vi "read report n write as formate sql.vi"(8 "error in":errorcluster, 10 "Table Name":string="Detailed_Report", 11 "file path (dialog if empty)":path) -> (0 "error out":errorcluster)   [LabVIEW 2017]
uses:
  <vilib>/Utility/file.llb/Read Delimited Spreadsheet (string).vi
panel:
  out "array w/ subset deleted":string[][](array[string])
  out "all rows":string[][](array[string])
  out "Serial Number":string
  in  "User Name 2":string="mmk"
  in  "Shift 2":string="A"
  in  "Test Type 2":string="Test type"
  in  "Excepted Value 2":string="Excepted Value"
  out "Application Verision":string
  out "Variant":string
  out "Model":string
  out "all rows 2":string[][](array[string])
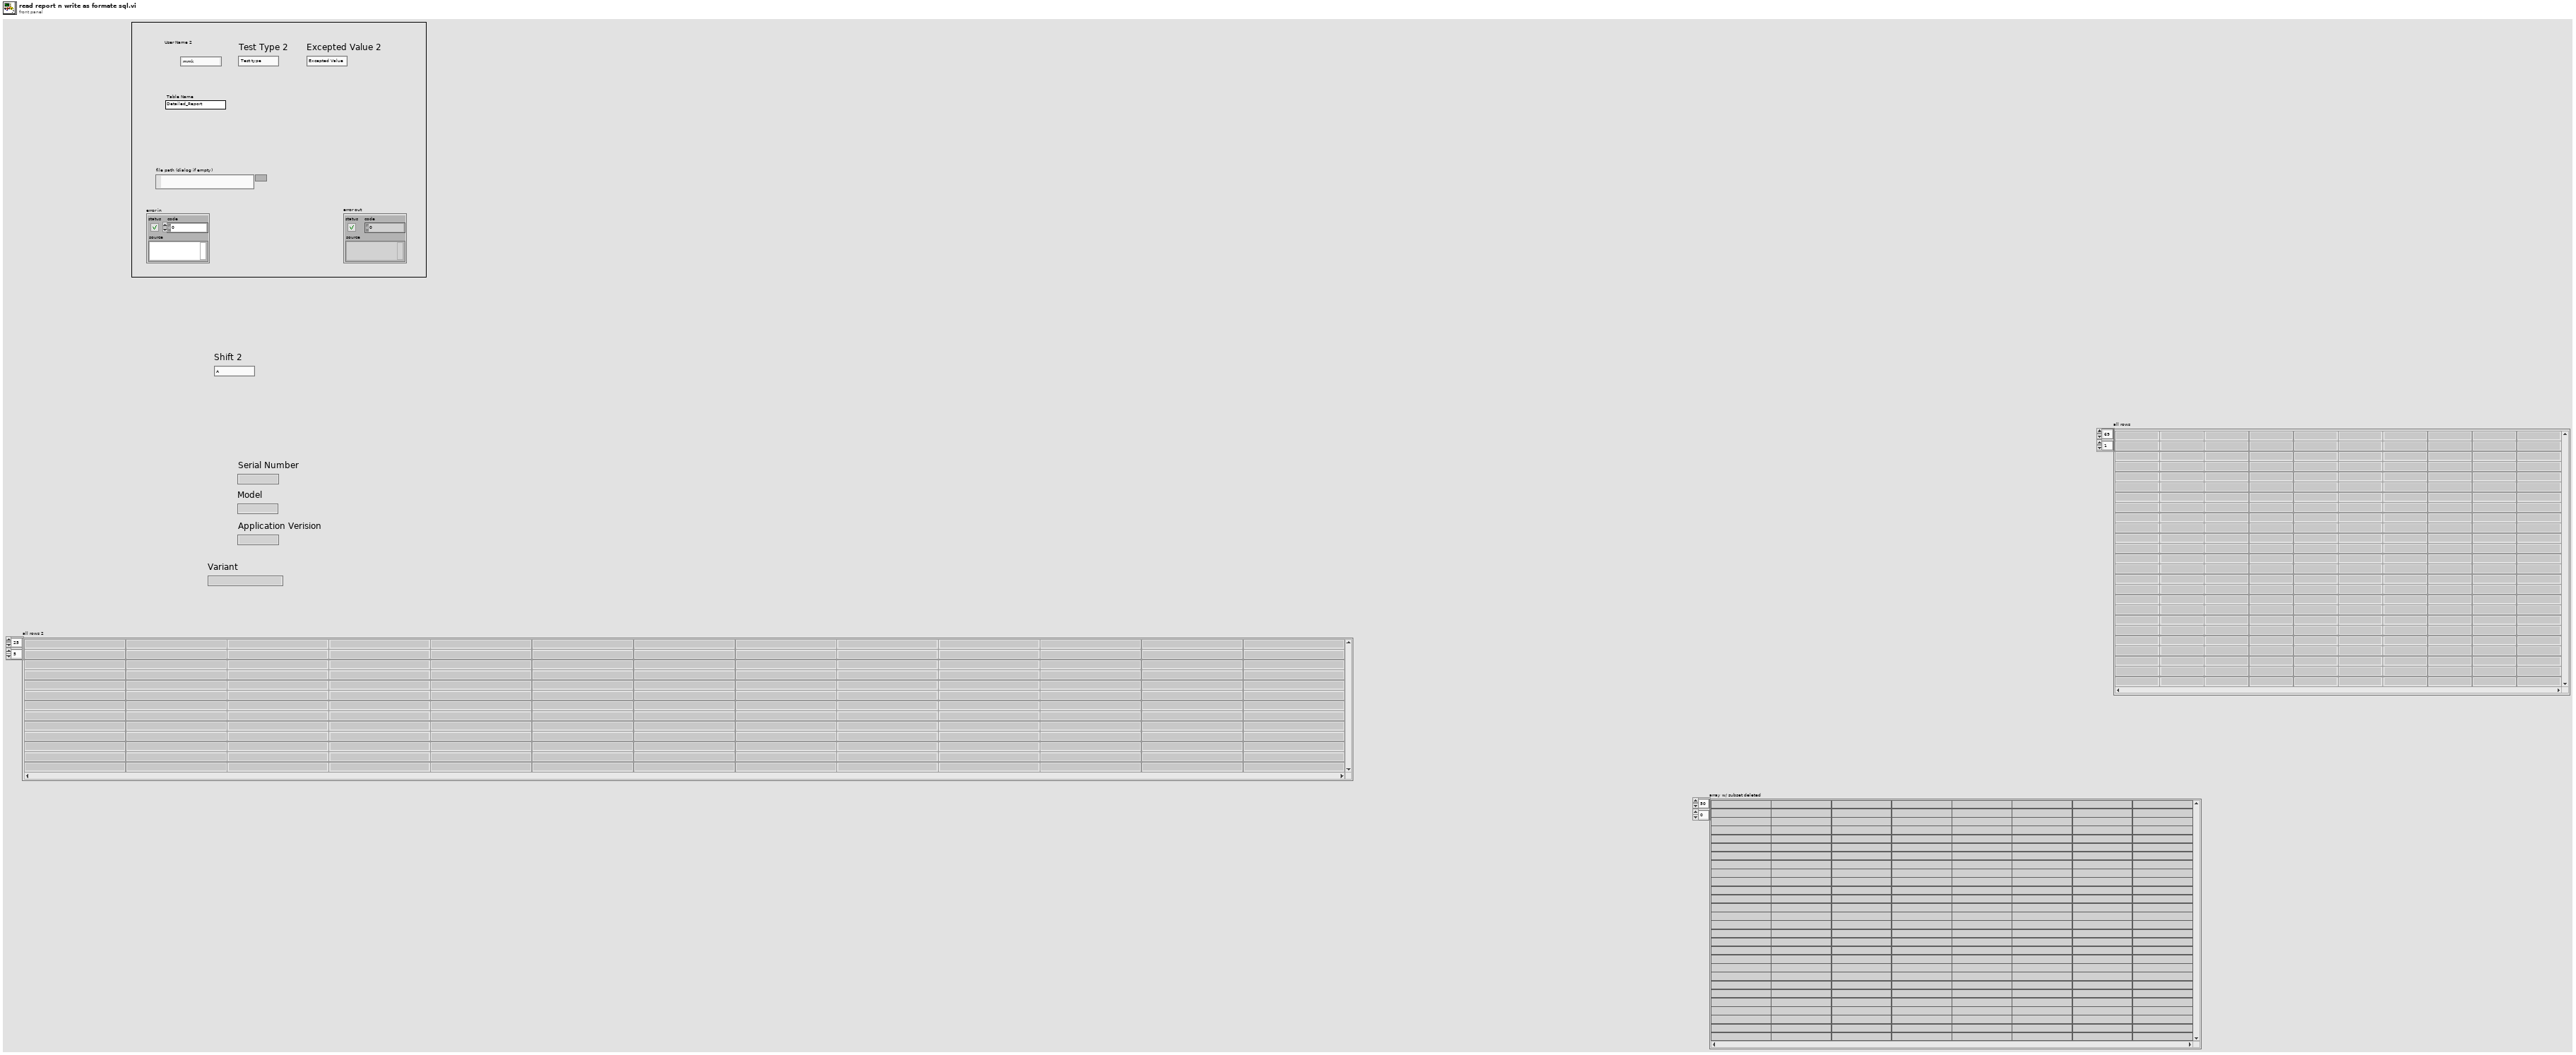
[diagram p1: front panel]
types:
  T1 = cluster{string, string, string, string, string, string, string, string, string, string, string, string, string, string, string}
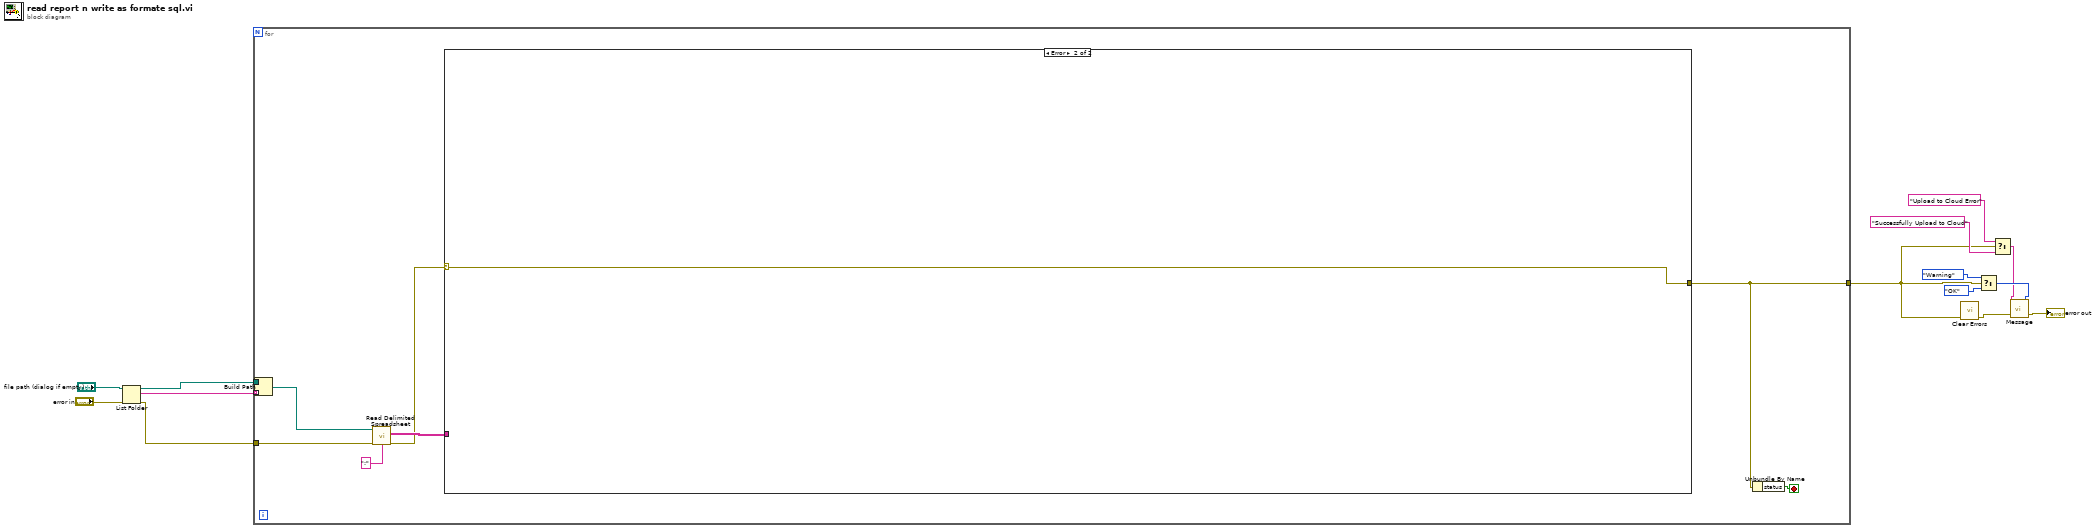
[diagram p0: block diagram]
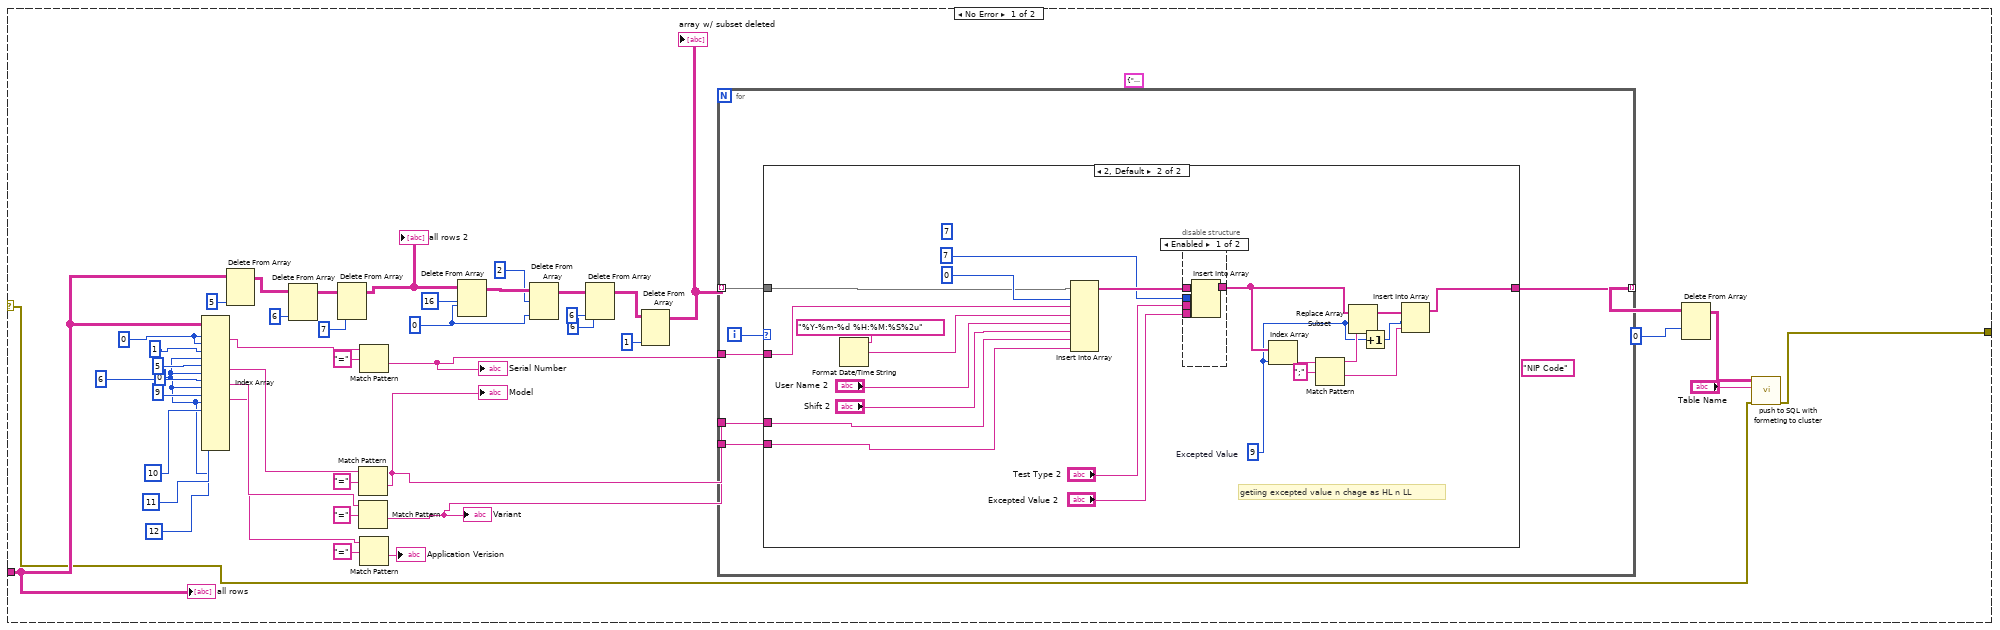
[diagram p2: hidden frame]
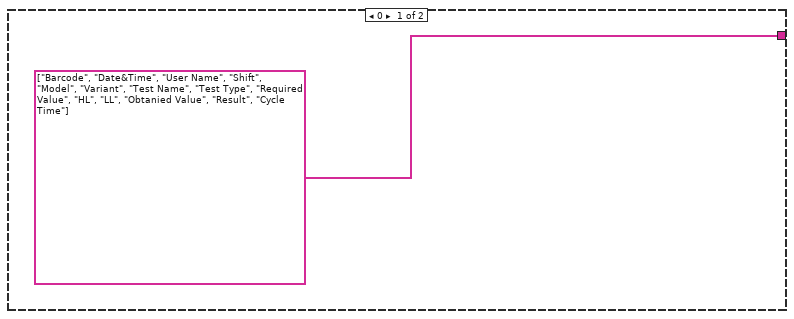
[diagram p3: hidden frame]
diagram:
  n1 = List Folder(path="file path (dialog if empty)", error in="error in") -> (path out=w12:path, filenames=w13:string[], error out=w1:errorcluster)  [unwired: 2 in, 1 out]
  n2 = for {
    tunnel: w13 -> [w19] mode=indexing
    tunnel: w12 -> [w20]
    tunnel: w1 -> [w17]
    tunnel: [w15] -> w6
    stop <- w16 stop-if-true
    n3 = Build Path(base path=w20, name or relative path=w19) -> (appended path=w18:path)
    n4 = call-poly <vilib>:"Read Delimited Spreadsheet.vi"("file path (dialog if empty)"=w18, "error in (no error)"=w17, "delimiter (\\t)"=":" ("delimiter (\\t)")) -> ("all rows"=w22:string[][], "error out"=w21:errorcluster)  [unwired: 7 in, 4 out]
    n5 = case shown="Error" w21 {
      selector: w21 -> [w26 w103]
      tunnel: w22 -> [w41 _]
      tunnel: [w24 w103] -> w15
      frame No Error {
        (unwired) T1 {"barcode", "2019-12-13 20:24:09.05", "1", "shifr", "model", "variant", "test name", "test type", "hl", "ll", "shifr", "obtained", "resrut", "Cycle time", "nip code"}
        w56 = 0 ("index (row)")
        w48 = 0 ("disabled index (col)")
        w37 = 0 ("disabled index (col)")
        n6 = Index Array(array=w41, index (row) #1=w56, index (col) #1=w56, index (row) #2=1 ("index (row)"), index (col) #2=w37, index (row) #3=5 ("index (row)"), index (col) #3=w37, index (row) #4=6 ("index (row)"), index (col) #4=w37, index (row) #5=9 ("index (row)"), index (col) #5=w37, index (row) #6=10 ("index (row)"), index (col) #6=w37, index (row) #7=11 ("index (row)"), index (col) #7=w37, index (row) #8=12 ("index (row)"), index (col) #8=w37) -> (element #1=w54:string, element #3=w66:string, element #4=w63:string, element #5=w59:string)  [unwired: 4 out]
        n7 = Delete From Array(array=w41, index (col)=5 ("disabled index (col)")) -> (array with subset deleted=w40:string[][])  [unwired: 2 in, 1 out]
        n8 = Delete From Array(array=w40, index (col)=6 ("disabled index (col)")) -> (array with subset deleted=w46:string[][])  [unwired: 2 in, 1 out]
        n9 = Delete From Array(array=w46, index (col)=7 ("disabled index (col)")) -> (array with subset deleted=w45:string[][])  [unwired: 2 in, 1 out]
        "all rows 2" <- w45
        n10 = Match Pattern(string=w66, regular expression="=") -> (after substring=w52:string)  [unwired: 1 in, 3 out]
        "Model" <- w52
        n11 = Match Pattern(string=w63, regular expression="=") -> (after substring=w51:string)  [unwired: 1 in, 3 out]
        "Variant" <- w51
        n12 = Match Pattern(string=w54, regular expression="=") -> (after substring=w53:string)  [unwired: 1 in, 3 out]
        "Serial Number" <- w53
        n13 = Match Pattern(string=w59, regular expression="=") -> (after substring=→"Application Verision":string)  [unwired: 1 in, 3 out]
        n14 = Delete From Array(array=w45, length=16, index (row)=w48) -> (array with subset deleted=w49:string[][])  [unwired: 1 in, 1 out]
        n15 = Delete From Array(array=w49, length=2, index (col)=w48) -> (array with subset deleted=w35:string[][])  [unwired: 1 in, 1 out]
        n16 = Delete From Array(array=w35, length=6, index (col)=6 ("disabled index (col)")) -> (array with subset deleted=w32:string[][])  [unwired: 1 in, 1 out]
        n17 = Delete From Array(array=w32, index (col)=1 ("disabled index (col)")) -> (array with subset deleted=w30:string[][])  [unwired: 2 in, 1 out]
        "array w/ subset deleted" <- w30
        n18 = for {
          tunnel: w30 -> [w73] mode=indexing
          tunnel: [w68] -> w28 mode=indexing
          tunnel: w53 -> [w71]
          tunnel: w52 -> [w70]
          tunnel: w51 -> [w69]
          i -> [w72]
          (unwired) "NIP Code" ("new element/subarray")
          n19 = case shown="2, Default" w72 {
            tunnel: w73 -> [_ w84]
            tunnel: [string[] ["Barcode", "Date&Time", "User Name", "Shift", "Model", "Variant", "Test Name", "Test Type", "Required Value", "HL", "LL", "Obtanied Value", "Result", "Cycle Time"] w75] -> w68
            tunnel: w71 -> [_ w87]
            tunnel: w70 -> [_ w86]
            tunnel: w69 -> [_ w85]
            frame 0 {
            }
            frame 2, Default {
              w78 = 9  # Excepted Value
              (unwired) 7 ("index")
              # "getiing excepted value n chage as HL n LL"
              n20 = Format Date/Time String(time format string (%c)="%Y-%m-%d %H:%M:%S%2u") -> (date/time string=w88:string)  [unwired: 2 in]
              n21 = Insert Into Array(array=w84, index=0, new element #1=w87, new element #2=w88, new element #3="User Name 2", new element #4="Shift 2", new element #5=w86, new element #6=w85) -> (w93:string[])
              n22 = disable-structure shown="Enabled" {
                disable-tunnel: w93 -> [w101 w102]
                disable-tunnel: 7 ("index") -> [w100 _]
                disable-tunnel: "Test Type 2" -> [w99 _]
                disable-tunnel: "Excepted Value 2" -> [w98 _]
                disable-tunnel: [w97 w102] -> w81
                frame Enabled {
                  n23 = Insert Into Array(array=w101, index=w100, new element #1=w99, new element #2=w98) -> (w97:string[])
                }
                frame Disabled {
                }
              }
              n24 = Index Array(array=w81, index=w78) -> (element=w83:string)
              n25 = Match Pattern(string=w83, regular expression=";") -> (before substring=w80:string, after substring=w76:string)  [unwired: 1 in, 2 out]
              n26 = Replace Array Subset(array=w81, new element=w80, index=w78) -> (w79:string[])
              n27 = Increment(x=w78) -> (x+1=w77:i32)
              n28 = Insert Into Array(array=w79, index=w77, new element=w76) -> (w75:string[])
            }
          }
        }
        n29 = Delete From Array(array=w28, index (row)=0 ("disabled index (col)")) -> (array with subset deleted=w27:string[][])  [unwired: 2 in, 1 out]
        n30 = call "push to SQL with formeting to cluster.vi"("error in (no error) 3"=w26, "Table Name"="Table Name", "array w/ subset deleted 2"=w27) -> ("error Out (no error) 2"=w24:errorcluster)  [unwired: 8 in]
        "all rows" <- w41
      }
      frame Error {
      }
    }
    n31 = Unbundle By Name(w15) -> ("status"=w16:bool)
  }
  n32 = call <vilib>:"Clear Errors.vi"("error in (no error)"=w6) -> ("error out"=w5:errorcluster)  [unwired: 5 in, 1 out]
  n33 = Select(t=enum16{"Error", "Warning", "OK"}."Warning" ("Enum"), s=w6, f=enum16{"Error", "Warning", "OK"}."OK" ("Enum")) -> (s? t:f=w4:enum16{"Error", "Warning", "OK"})
  n34 = Select(t="Upload to Cloud Error" ("Message"), s=w6, f="Successfully Upload to Cloud" ("Message")) -> (s? t:f=w3:string)
  n35 = call "Message.vi"("Enum"=w4, "error in (no error)"=w5, "Message"=w3) -> ("error out"=→"error out":errorcluster)  [unwired: 1 in, 1 out]
